vi "Example Graph.vi"() -> ()   [LabVIEW 2010]
uses:
  C:/tf/play/labview/Tinkerforge.dll
  Tinkerforge.dll
panel:
  in  "stop":bool
  out "graph":i32[](graph)
  in  "uid":string="8e7"
  in  "port":i32=4223
  in  "host":string="localhost"
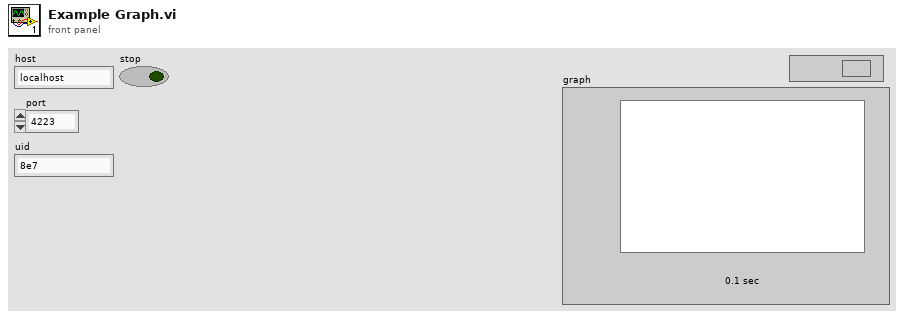
[diagram p1: front panel]
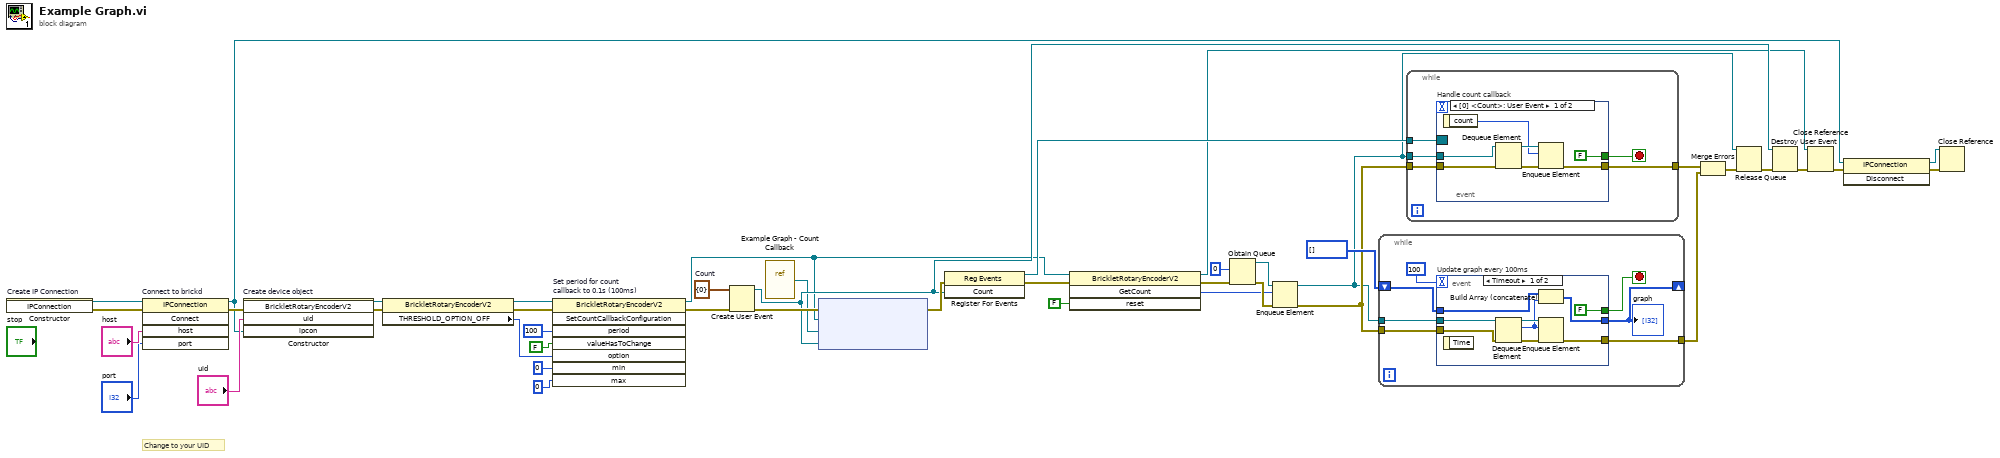
[diagram p0: block diagram]
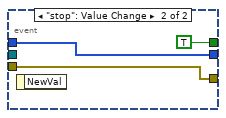
[diagram p2: hidden frame]
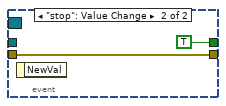
[diagram p3: hidden frame]
diagram:
  w29 = cluster{"count":i32} {"count"=0}  # Count
  # "Change to your UID"
  n1 = constructor on="Create IP Connection" class="IPConnection"() -> (reference out=w43:refnum<k24>, error out=w16:errorcluster)  [unwired: 3 in, 1 out]
  n2 = invoke on="Connect to brickd" class="IPConnection" method="Connect"(reference=w43, error in=w16, "host"="host", "port"="port") -> (reference out=w36:refnum<k24>, error out=w39:errorcluster)  [unwired: 1 in, 3 out]
  n3 = constructor on="Create device object" class="BrickletRotaryEncoderV2"(error in=w39, "uid"="uid", "ipcon"=w36) -> (reference out=w6:refnum<k24>, error out=w3:errorcluster)  [unwired: 2 in, 3 out]
  n4 = property class="BrickletRotaryEncoderV2"(reference=w6, error in=w3) -> (reference out=w5:refnum<k24>, error out=w2:errorcluster, "THRESHOLD_OPTION_OFF"=w4:u16)
  n5 = invoke on="Set period for count\ncallback to 0.1s (100ms)" class="BrickletRotaryEncoderV2" method="SetCountCallbackConfiguration"(reference=w5, error in=w2, "period"=i64 100, "valueHasToChange"=FALSE, "option"=w4, "min"=0, "max"=0) -> (reference out=w13:refnum<k24>, error out=w28:errorcluster)  [unwired: 1 in, 6 out]
  n6 = Create User Event(user event datatype=w29, error in=w28) -> (user event=w31:refnum<user-event>, error out=w34:errorcluster)
  n7 = vi-ref "Example Graph - Count Callback.vi"() -> ("vi reference"=w1:refnum<vi>)
  n8 = node ("Register Event Callback")(w34, w13, w1, w31) -> (w33:errorcluster)  [unwired: 1 in, 1 out]
  n9 = register-events(error in=w33, w31) -> (reference out=w32:refnum<event-registration>, error out=w15:errorcluster)  [unwired: 1 in]
  n10 = invoke class="BrickletRotaryEncoderV2" method="GetCount"(reference=w13, error in=w15, "reset"=FALSE) -> (reference out=w12:refnum<k24>, error out=w14:errorcluster, "GetCount"=w11:i32)  [unwired: 1 in, 1 out]
  n11 = Obtain Queue(element data type=0, error in (no error)=w14) -> (queue out=w20:refnum<queue>, error out=w22:errorcluster)  [unwired: 3 in, 1 out]
  n12 = Enqueue Element(queue=w20, element=w11, error in (no error)=w22) -> (queue out=w17:refnum<queue>, error out=w21:errorcluster)  [unwired: 1 in, 1 out]
  n13 = while {
    tunnel: [w46] -> w26
    tunnel: w21 -> [w47]
    shift-right: [w48] -> _
    shift-left: i32[] [] -> [w49]
    tunnel: w17 -> [w45]
    stop <- w44 stop-if-true
    n14 = event "Update graph every 100ms" shown="[0] Timeout" {
      selector: _ -> [_ _]
      dyn-events: _ -> [_ _]
      timeout: 100 -> [_ _]
      tunnel: [w59 w61] -> w48
      tunnel: w49 -> [w52 w61]
      tunnel: w47 -> [w58 w60]
      tunnel: [w55 w60] -> w46
      tunnel: w45 -> [w57 _]
      tunnel: [FALSE TRUE] -> w44
      event Timeout {
        n15 = event-data() -> ()  [unwired: 1 in, 1 out]
        n16 = Dequeue Element(queue=w57, error in (no error)=w58) -> (queue out=w54:refnum<queue>, element=w53:i32, error out=w56:errorcluster)  [unwired: 1 in, 1 out]
        n17 = Build Array (concatenate)(w52, w53) -> (w59:i32[])
        n18 = Enqueue Element(queue=w54, element=w53, error in (no error)=w56) -> (error out=w55:errorcluster)  [unwired: 1 in, 2 out]
      }
      event "stop": Value Change {
        n19 = event-data() -> ()  [unwired: 1 in, 1 out]
      }
    }
    "graph" <- w48
  }
  n20 = while {
    tunnel: w32 -> [w67]
    tunnel: [w65] -> w25
    tunnel: w21 -> [w66]
    tunnel: w17 -> [w64]
    stop <- w63 stop-if-true
    n21 = event "Handle count callback" shown="[0] <Count>: User Event" {
      selector: w67 -> [_ _]
      dyn-events: _ -> [_ _]
      timeout: _ -> [_ _]
      tunnel: w66 -> [w74 w75]
      tunnel: [w72 w75] -> w65
      tunnel: w64 -> [w71 _]
      tunnel: [FALSE TRUE] -> w63
      event User Event {
        n22 = event-data() -> ("count"=w68:i32)  [unwired: 1 in]
        n23 = Dequeue Element(queue=w71, error in (no error)=w74) -> (queue out=w70:refnum<queue>, error out=w73:errorcluster)  [unwired: 1 in, 2 out]
        n24 = Enqueue Element(queue=w70, element=w68, error in (no error)=w73) -> (error out=w72:errorcluster)  [unwired: 1 in, 2 out]
      }
      event "stop": Value Change {
        n25 = event-data() -> ()  [unwired: 1 in, 1 out]
      }
    }
  }
  n26 = Merge Errors(w25, w26) -> (w19:errorcluster)
  n27 = Release Queue(queue=w17, error in (no error)=w19) -> (error out=w18:errorcluster)  [unwired: 1 in, 2 out]
  n28 = Destroy User Event(user event=w31, error in=w18) -> (error out=w30:errorcluster)
  n29 = Close Reference(reference=w12, error in (no error)=w30) -> (error out=w38:errorcluster)
  n30 = invoke class="IPConnection" method="Disconnect"(reference=w36, error in=w38) -> (reference out=w35:refnum<k24>, error out=w37:errorcluster)  [unwired: 1 in, 1 out]
  n31 = Close Reference(reference=w35, error in (no error)=w37) -> ()  [unwired: 1 out]
